vi "DDS Timeout Check.vi"(8 "error in (no error)":errorcluster, 11 "DDS Settings":T1={"Enable DDS"=TRUE, "Array of DDS Boxes"=[{"DDS box device reference"={"NI USB-8451 device reference"="USB0::0x3923::0x7166::01574F57::RAW", "DIO port"=0, "Serial Clock Rate [kHz]"=1000}, "Array of DDS Channels (4)"=[{"Power"=FALSE, "Channel Parameters"={"Ref Clock Rate [kHz]"=1000.0, "Full Scale Output\nPower [dBm]"=0.0}, "RAM Enable"=FALSE, "RAM Dest Type"=0, "RAM Default"={"Frequency [MHz]"=0.0, "Amplitude [dBm]"=0.0, "Phase Offset [rad]"=0.0}, "Array of DDS Profiles (8)"=[], "description"=""}, {"Power"=FALSE, "Channel Parameters"={"Ref Clock Rate [kHz]"=1000.0, "Full Scale Output\nPower [dBm]"=0.0}, "RAM Enable"=FALSE, "RAM Dest Type"=0, "RAM Default"={"Frequency [MHz]"=0.0, "Amplitude [dBm]"=0.0, "Phase Offset [rad]"=0.0}, "Array of DDS Profiles (8)"=[], "description"=""}, {"Power"=FALSE, "Channel Parameters"={"Ref Clock Rate [kHz]"=1000.0, "Full Scale Output\nPower [dBm]"=0.0}, "RAM Enable"=FALSE, "RAM Dest Type"=0, "RAM Default"={"Frequency [MHz]"=0.0, "Amplitude [dBm]"=0.0, "Phase Offset [rad]"=0.0}, "Array of DDS Profiles (8)"=[], "description"=""}, {"Power"=FALSE, "Channel Parameters"={"Ref Clock Rate [kHz]"=1000.0, "Full Scale Output\nPower [dBm]"=0.0}, "RAM Enable"=FALSE, "RAM Dest Type"=0, "RAM Default"={"Frequency [MHz]"=0.0, "Amplitude [dBm]"=0.0, "Phase Offset [rad]"=0.0}, "Array of DDS Profiles (8)"=[], "description"=""}], "Enable"=TRUE, "description"=""}, {"DDS box device reference"={"NI USB-8451 device reference"="USB0::0x3923::0x7166::01574FA5::RAW", "DIO port"=0, "Serial Clock Rate [kHz]"=1000}, "Array of DDS Channels (4)"=[{"Power"=FALSE, "Channel Parameters"={"Ref Clock Rate [kHz]"=1000.0, "Full Scale Output\nPower [dBm]"=0.0}, "RAM Enable"=FALSE, "RAM Dest Type"=0, "RAM Default"={"Frequency [MHz]"=0.0, "Amplitude [dBm]"=0.0, "Phase Offset [rad]"=0.0}, "Array of DDS Profiles (8)"=[], "description"=""}, {"Power"=FALSE, "Channel Parameters"={"Ref Clock Rate [kHz]"=1000.0, "Full Scale Output\nPower [dBm]"=0.0}, "RAM Enable"=FALSE, "RAM Dest Type"=0, "RAM Default"={"Frequency [MHz]"=0.0, "Amplitude [dBm]"=0.0, "Phase Offset [rad]"=0.0}, "Array of DDS Profiles (8)"=[], "description"=""}, {"Power"=FALSE, "Channel Parameters"={"Ref Clock Rate [kHz]"=1000.0, "Full Scale Output\nPower [dBm]"=0.0}, "RAM Enable"=FALSE, "RAM Dest Type"=0, "RAM Default"={"Frequency [MHz]"=0.0, "Amplitude [dBm]"=0.0, "Phase Offset [rad]"=0.0}, "Array of DDS Profiles (8)"=[], "description"=""}, {"Power"=FALSE, "Channel Parameters"={"Ref Clock Rate [kHz]"=1000.0, "Full Scale Output\nPower [dBm]"=0.0}, "RAM Enable"=FALSE, "RAM Dest Type"=0, "RAM Default"={"Frequency [MHz]"=0.0, "Amplitude [dBm]"=0.0, "Phase Offset [rad]"=0.0}, "Array of DDS Profiles (8)"=[], "description"=""}], "Enable"=TRUE, "description"=""}, {"DDS box device reference"={"NI USB-8451 device reference"="USB0::0x3923::0x7166::01574F73::RAW", "DIO port"=0, "Serial Clock Rate [kHz]"=1000}, "Array of DDS Channels (4)"=[{"Power"=FALSE, "Channel Parameters"={"Ref Clock Rate [kHz]"=1000.0, "Full Scale Output\nPower [dBm]"=0.0}, "RAM Enable"=FALSE, "RAM Dest Type"=0, "RAM Default"={"Frequency [MHz]"=0.0, "Amplitude [dBm]"=0.0, "Phase Offset [rad]"=0.0}, "Array of DDS Profiles (8)"=[], "description"=""}, {"Power"=FALSE, "Channel Parameters"={"Ref Clock Rate [kHz]"=1000.0, "Full Scale Output\nPower [dBm]"=0.0}, "RAM Enable"=FALSE, "RAM Dest Type"=0, "RAM Default"={"Frequency [MHz]"=0.0, "Amplitude [dBm]"=0.0, "Phase Offset [rad]"=0.0}, "Array of DDS Profiles (8)"=[], "description"=""}, {"Power"=FALSE, "Channel Parameters"={"Ref Clock Rate [kHz]"=1000.0, "Full Scale Output\nPower [dBm]"=0.0}, "RAM Enable"=FALSE, "RAM Dest Type"=0, "RAM Default"={"Frequency [MHz]"=0.0, "Amplitude [dBm]"=0.0, "Phase Offset [rad]"=0.0}, "Array of DDS Profiles (8)"=[], "description"=""}, {"Power"=FALSE, "Channel Parameters"={"Ref Clock Rate [kHz]"=1000.0, "Full Scale Output\nPower [dBm]"=0.0}, "RAM Enable"=FALSE, "RAM Dest Type"=0, "RAM Default"={"Frequency [MHz]"=0.0, "Amplitude [dBm]"=0.0, "Phase Offset [rad]"=0.0}, "Array of DDS Profiles (8)"=[], "description"=""}], "Enable"=TRUE, "description"=""}]} {"Array of DDS Boxes"."Array of DDS Channels (4)"."Channel Parameters"."Ref Clock Rate [kHz]" min=0.0}) -> (0 "error out":errorcluster, 3 "DDS Comms OK?":bool)   [LabVIEW 2013, in "DDS.lvclass"]
uses:
  cesium_controller/DDS/DDS.lvclass
  cesium_controller/DDS/DDS_Settings_Cluster.ctl
  Array_of_DDS_Boxes.ctl
  DDS_box_cluster.ctl
  DDS_box_device_reference.ctl
  <vilib>/ni845x/ni845x.llb/ni845xControl.ctl
  array_of_DDS_channels.ctl
  DDS_channel.ctl
  array_of_DDS_profiles.ctl
  DDS_profile.ctl
  DDS RAM mode.ctl
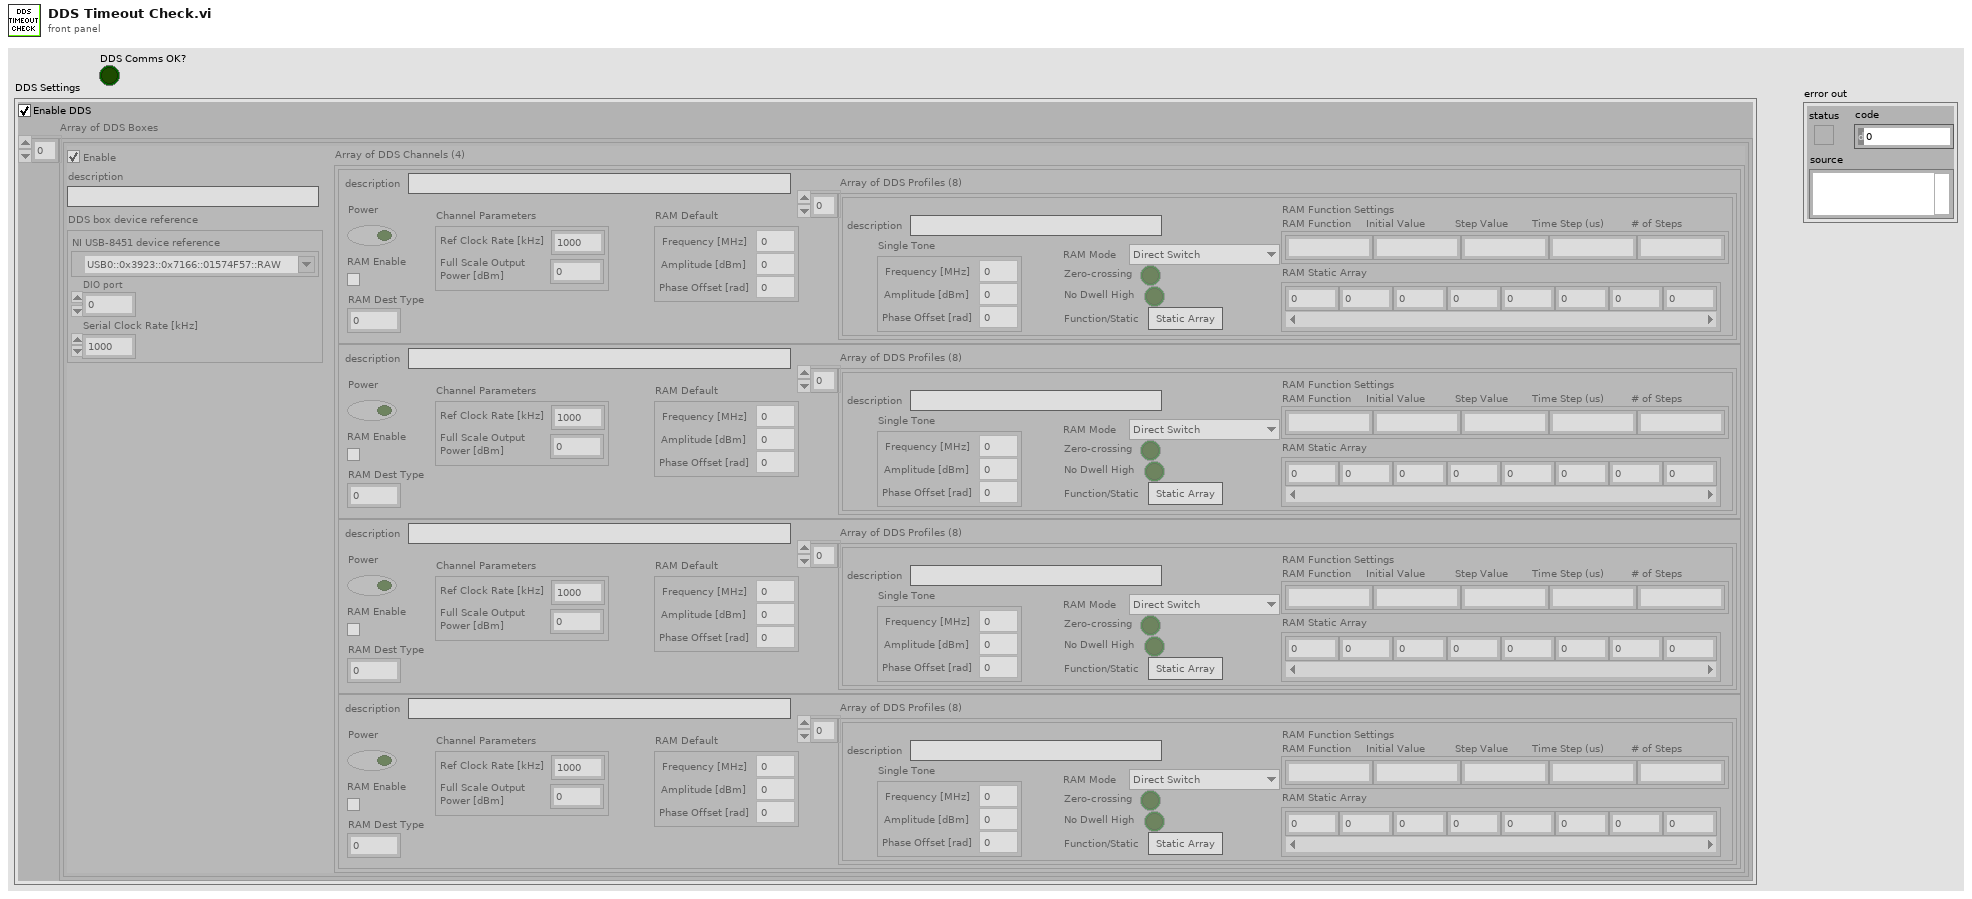
[diagram p1: front panel]
types:
  T1 = typedef "DDS_Settings_Cluster.ctl" = cluster{"Enable DDS":bool, "Array of DDS Boxes":T2}
  T2 = typedef "Array_of_DDS_Boxes.ctl" = T3[]
  T3 = typedef "DDS_box_cluster.ctl" = cluster{"DDS box device reference":T4, "Array of DDS Channels (4)":T6, "Enable":bool, "description":string}
  T4 = typedef "DDS_box_device_reference.ctl" = cluster{"NI USB-8451 device reference":T5, "DIO port":u8, "Serial Clock Rate [kHz]":u16}
  T5 = typedef "ni845xControl.ctl" = refnum<k21>
  T6 = typedef "DDS.lvclass/array_of_DDS_channels.ctl" = T7[]
  T7 = typedef "DDS.lvclass/DDS_channel.ctl" = cluster{"Power":bool, "Channel Parameters":cluster{"Ref Clock Rate [kHz]":dbl, "Full Scale Output\nPower [dBm]":dbl}, "RAM Enable":bool, "RAM Dest Type":u8, "RAM Default":cluster{"Frequency [MHz]":dbl, "Amplitude [dBm]":dbl, "Phase Offset [rad]":dbl}, "Array of DDS Profiles (8)":T8, "description":string}
  T8 = typedef "DDS.lvclass/array_of_DDS_profiles.ctl" = T9[]
  T9 = typedef "DDS_profile.ctl" = cluster{"Single Tone":cluster{"Frequency [MHz]":dbl, "Amplitude [dBm]":dbl, "Phase Offset [rad]":dbl}, "RAM Mode ":T10, "Zero-crossing":bool, "No Dwell High":bool, "Function/Static":bool, "RAM Function Settings":string[], "RAM Static Array":dbl[], "description":string}
  T10 = typedef "DDS RAM mode.ctl" = enum16{"Direct Switch", "Ramp Up", "Bidirectional Ramp", "Continuous Bidirectional Ramp", "Continuous Recirculate", "Direct Switch 2", "Direct Switch 3", "Direct Switch 4"}
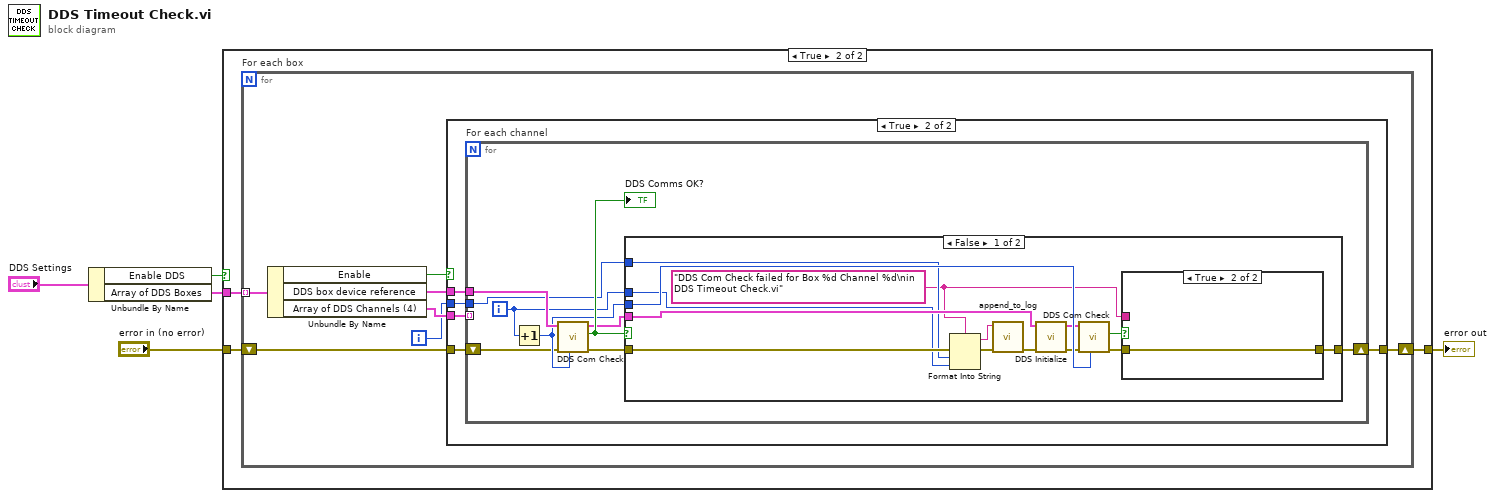
[diagram p0: block diagram]
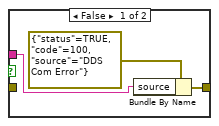
[diagram p4: hidden frame]
diagram:
  n1 = Unbundle By Name("DDS Settings") -> ("Enable DDS"=w4:bool, "Array of DDS Boxes"=w3:T2)
  n2 = case shown="True" w4 {
    tunnel: w3 -> [_ w9]
    tunnel: "error in (no error)" -> [w6 w8]
    tunnel: [w6 w7] -> w1
    frame False {
    }
    frame True {
      n3 = for "For each box" {
        tunnel: w9 -> [w16] mode=indexing
        shift-right: [w12] -> w7
        shift-left: w8 -> [w13]
        i -> [w10]
        n4 = Unbundle By Name(w16) -> ("Enable"=w14:bool, "DDS box device reference"=w15:T4, "Array of DDS Channels (4)"=w11:T6)
        n5 = case shown="True" w14 {
          tunnel: w15 -> [_ w22]
          tunnel: w13 -> [w17 w21]
          tunnel: [w17 w20] -> w12
          tunnel: w11 -> [_ w19]
          tunnel: w10 -> [_ w18]
          frame False {
          }
          frame True {
            n6 = for "For each channel" {
              tunnel: w22 -> [w31]
              shift-right: [w27] -> w20
              shift-left: w21 -> [w24]
              tunnel: w19 -> [_] mode=indexing
              tunnel: w18 -> [w23]
              i -> [w26]
              n7 = Increment(x=w26) -> (x+1=w25:i32)
              n8 = call "DDS Com Check.vi"("channel number (1)"=w25, "error in (no error)"=w24, "DDS ref in"=w31) -> ("error out"=w28:errorcluster, "Passed?"=w30:bool, "DDS ref out"=w29:T4)  [unwired: 4 in]
              "DDS Comms OK?" <- w30
              n9 = case shown="False" w30 {
                tunnel: w29 -> [w45 _]
                tunnel: w28 -> [w43 w50]
                tunnel: [w44 w50] -> w27
                tunnel: w26 -> [w34 _]
                tunnel: w25 -> [w42 _]
                tunnel: w23 -> [w33 _]
                frame False {
                  w32 = "DDS Com Check failed for Box %d Channel %d\nin DDS Timeout Check.vi" ("format string")
                  n10 = Format Into String(format string=w32, error in=w43, w33, w34) -> (resulting string=w41:string, error out=w40:errorcluster)  [unwired: 1 in]
                  n11 = call "append_to_log.vi"("error in"=w40, "string"=w41) -> ("error out"=w39:errorcluster)  [unwired: 9 in]
                  n12 = call "DDS Initialize.vi"("error in (no error)"=w39, "DDS ref in"=w45) -> ("error out"=w37:errorcluster, "DDS ref out"=w38:T4)  [unwired: 8 in]
                  n13 = call "DDS Com Check.vi"("channel number (1)"=w42, "error in (no error)"=w37, "DDS ref in"=w38) -> ("error out"=w35:errorcluster, "Passed?"=w36:bool)  [unwired: 4 in, 1 out]
                  n14 = case shown="True" w36 {
                    tunnel: [w46 w49] -> w44
                    tunnel: w35 -> [_ w49]
                    tunnel: w32 -> [w48 _]
                    frame False {
                      n15 = Bundle By Name(cluster=errorcluster {"status"=TRUE, "code"=100, "source"="DDS Com Error"} ("error out"), "source"=w48) -> (w46:errorcluster)
                    }
                    frame True {
                    }
                  }
                }
                frame True {
                }
              }
            }
          }
        }
      }
    }
  }
  "error out" <- w1
